vi "UART Open Device.vi"(8 "error in (no error)":errorcluster, 10 "Reserved":i32, 11 "DevIndex":i32) -> (0 "error out":errorcluster, 3 "function return":i32)   [LabVIEW 2012, in "ControlUART.lvlib"]
doc: "int WINAPI UART_OpenDevice(int DevIndex,int Reserved);"
uses:
  ControlUART.lvlib
  Ginkgo_Driver.dll
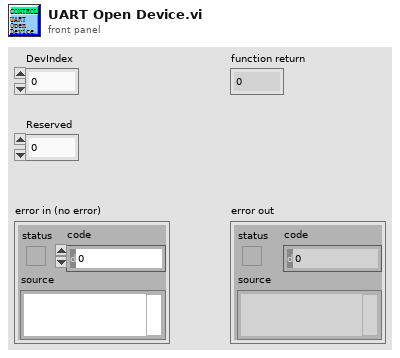
[diagram p1: front panel]
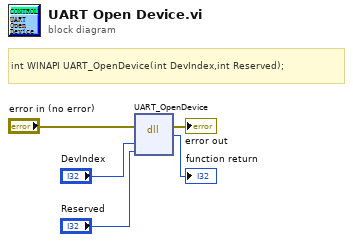
[diagram p0: block diagram]
diagram:
  # "int WINAPI UART_OpenDevice(int DevIndex,int Reserved);"
  n1 = dll-call lib="E:/Project/vt_ginkgo/truck/Ginkgo Driver/vs2010/Ginkgo_USB-I2C_API_v2.0.3.0/lib/labview_32bit/ControlUART/Ginkgo_Driver.*" fn="UART_OpenDevice"(error in="error in (no error)", "DevIndex"="DevIndex", "Reserved"="Reserved") -> (error out=→"error out":errorcluster, →"function return":i32)  [unwired: 4 in, 1 out]
